vi "Comparison_Decision.vi"(9 "decision":dbl[](array[numeric]), 10 "SWLDA":dbl[](array[numeric]), 11 "EPR_발생_total":i16[](array[numeric])) -> (3 "selected":i32)   [LabVIEW 2014]
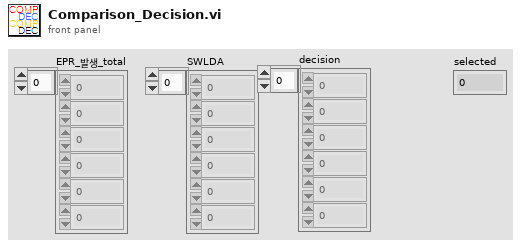
[diagram p1: front panel]
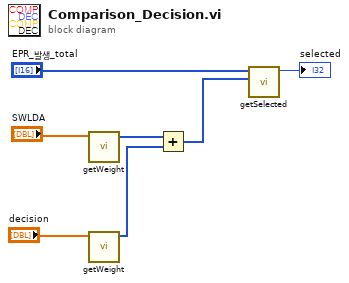
[diagram p0: block diagram]
diagram:
  n1 = call "getWeight.vi"("Array"="SWLDA") -> ("Weight"=w5:i32[])  [unwired: 10 in]
  n2 = call "getWeight.vi"("Array"="decision") -> ("Weight"=w4:i32[])  [unwired: 10 in]
  n3 = Add(x=w5, y=w4) -> (x+y=w2:i32[])
  n4 = call "getSelected.vi"("Weight"=w2, "Predict"="EPR_발생_total") -> ("selected"=→"selected":i32)  [unwired: 9 in]
